vi "Read External Payload.vi"(8 "error in (no error)":errorcluster, 9 "Timeout (ms)":i32, 10 "Data in":u8[](array[numeric]), 11 "CIFFIFO in":refnum<class "CIF_CIPC_Fifo_U8.lvclass">) -> (0 "error out":errorcluster, 1 "timed out?":bool, 2 "Data out":u8[](array[numeric]), 3 "CIFFIFO out":refnum<class "CIF_CIPC_Fifo_U8.lvclass">, 4 "Header":T1)   [LabVIEW 2021, in "CIF_CIPC_Fifo_U8.lvclass"]
doc: "Read the full payload bytes, including the encoded header. This is intended for advanced applications where the full buffer will be sent externally."
uses:
  CIF_CIPC_Fifo_U8.lvclass
  CIF_CIPC_Fifo_U8.lvclass/CIF_CIPC_Fifo_U8.ctl
  ChannelCommon/typedef/FIFO Header.ctl
  ChannelCommon/ChannelCommon.lvlib
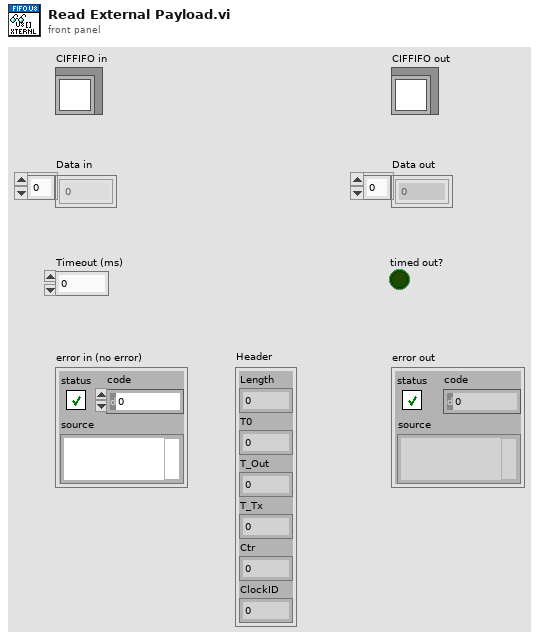
[diagram p1: front panel]
types:
  T1 = typedef "ChannelCommon.lvlib/FIFO Header.ctl" = cluster{"Length":u64, "T0":i64, "T_Out":i64, "T_Tx":i64, "Ctr":u64, "ClockID":u8}
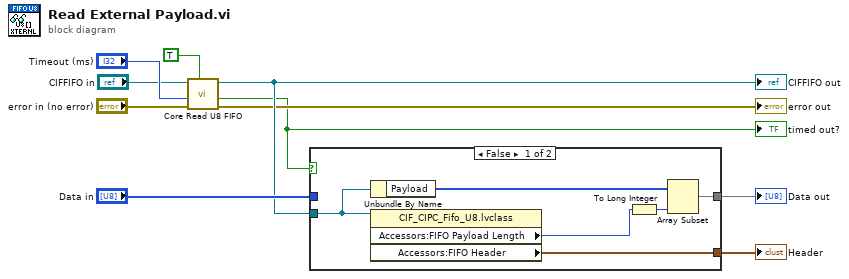
[diagram p0: block diagram]
diagram:
  n1 = call "Core Read U8 FIFO.vi"("Include Header"=TRUE, "error in (no error)"="error in (no error)", "Timeout (ms)"="Timeout (ms)", "CIFFIFO in"="CIFFIFO in") -> ("error out"=→"error out":errorcluster, "timed out?"=w2:bool, "CIFFIFO out"=w4:refnum<class "CIF_CIPC_Fifo_U8.lvclass">)  [unwired: 5 in]
  "timed out?" <- w2
  "CIFFIFO out" <- w4
  n2 = case shown="False" w2 {
    tunnel: w4 -> [w16 _]
    tunnel: [w14 w17] -> w6
    tunnel: [w13 _] -> w7
    tunnel: "Data in" -> [_ w17]
    frame False {
      n3 = Unbundle By Name(w16) -> ("Payload"=w15:u8[])
      n4 = property class="CIF_CIPC_Fifo_U8.lvclass"(reference=w16) -> ("Accessors:FIFO Payload Length"=w11:u64, "Accessors:FIFO Header"=w13:T1)  [unwired: 1 in, 2 out]
      n5 = To Long Integer(number=w11) -> (32bit integer=w12:i32)
      n6 = Array Subset(array=w15, length=w12) -> (w14:u8[])  [unwired: 1 in]
    }
    frame True {
    }
  }
  "Header" <- w7
  "Data out" <- w6
